vi "Register Events.vi"(8 "error in (no error)":errorcluster, 11 "Recipe Window in":refnum<class "Recipe Window.lvclass">) -> (0 "error out":errorcluster, 3 "Recipe Window out":refnum<class "Recipe Window.lvclass">, 5 "Pnl Events":refnum<event-registration>)   [LabVIEW 2021, in "Recipe.lvlib" / "Recipe Window.lvclass"]
uses:
  Recipe Window.lvclass
  Typedefs/Events--cluster.ctl
  Recipe Window.lvclass/Recipe Window.ctl
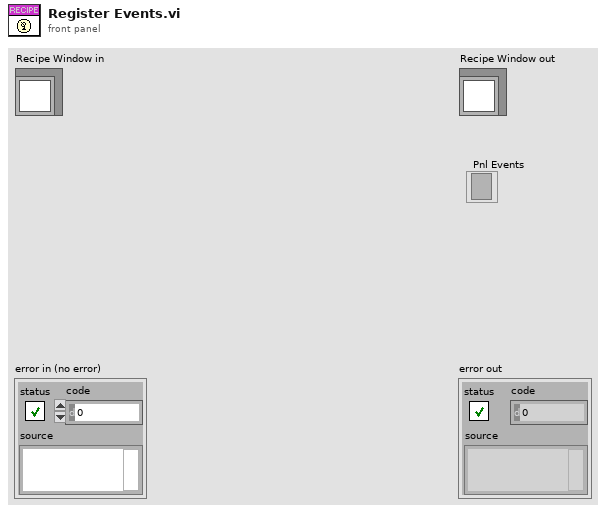
[diagram p1: front panel]
types:
  T1 = typedef "Recipe.lvlib/Recipe Window.lvclass/Events--cluster.ctl" = cluster{"Recipe Label New Value":refnum<user-event>}
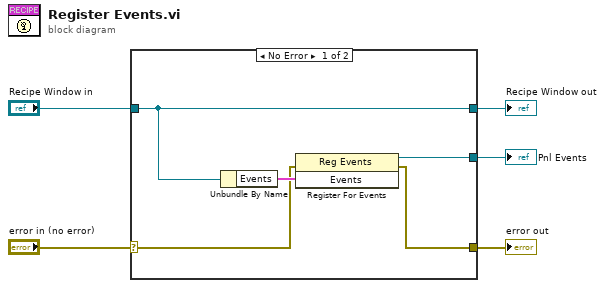
[diagram p0: block diagram]
diagram:
  n1 = case shown="No Error" "error in (no error)" {
    selector: "error in (no error)" -> [w8 w12]
    tunnel: [w7 w12] -> w4
    tunnel: [w9 w11] -> w2
    tunnel: "Recipe Window in" -> [w9 w11]
    tunnel: [w6 _] -> w1
    frame No Error {
      n2 = Unbundle By Name(w9) -> ("Events"=w10:T1)
      n3 = register-events(error in=w8, w10) -> (reference out=w6:refnum<event-registration>, error out=w7:errorcluster)  [unwired: 1 in]
    }
    frame Error {
    }
  }
  "error out" <- w4
  "Recipe Window out" <- w2
  "Pnl Events" <- w1
